vi "face rotate F+.vi"(8 "error in (no error)":errorcluster, 11 "cube in":T1) -> (0 "error out":errorcluster, 3 "cube out":T1)   [LabVIEW 2011]
uses:
  Typedef/cube.ctl
  Typedef/face.ctl
  Typedef/slice type.ctl
  Typedef/face rotate direction.ctl
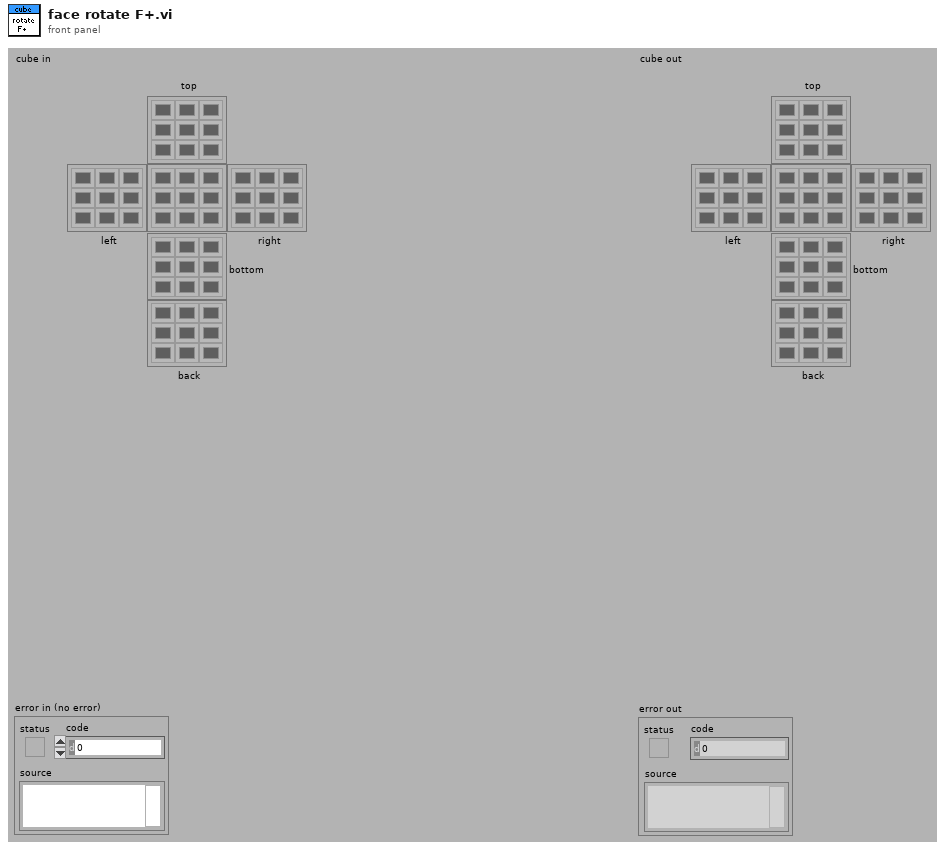
[diagram p1: front panel]
types:
  T1 = typedef "cube.ctl" = cluster{"top":T2, "left":T2, "right":T2, "bottom":T2, "back":T2, "front":T2}
  T2 = typedef "face.ctl" = u32[][]
  T3 = typedef "face rotate direction.ctl" = enum16{"+", "-"}
  T4 = typedef "slice type.ctl" = enum16{"row", "col"}
  T5 = typedef "slice.ctl" = u32[]
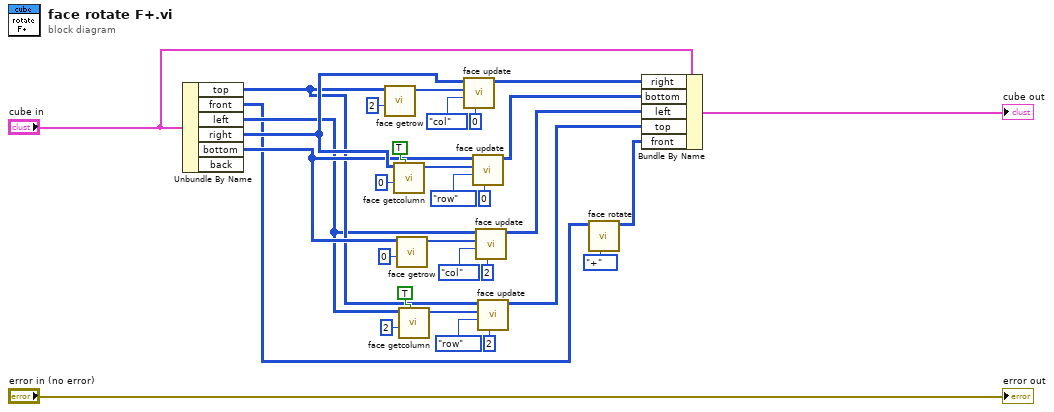
[diagram p0: block diagram]
diagram:
  n1 = Unbundle By Name("cube in") -> ("top"=w9:T2, "front"=w6:T2, "left"=w8:T2, "right"=w24:T2, "bottom"=w16:T2)  [unwired: 1 out]
  n2 = call "face getrow.vi"("row number"=u8 2, "face in"=w9) -> ("slice"=w30:T5)  [unwired: 8 in, 1 out]
  n3 = call "face getcolumn.vi"("reverse? (F)"=TRUE, "slice number"=u8 0 ("row number"), "face in"=w24) -> ("slice"=w22:T5)  [unwired: 7 in, 1 out]
  n4 = call "face getrow.vi"("row number"=u8 0, "face in"=w16) -> ("slice"=w20:T5)  [unwired: 8 in, 1 out]
  n5 = call "face getcolumn.vi"("reverse? (F)"=TRUE, "slice number"=u8 2 ("row number"), "face in"=w8) -> ("slice"=w10:T5)  [unwired: 7 in, 1 out]
  n6 = call "face update.vi"("slice number"=u8 0, "slice type"=slice_type."col", "slice"=w30, "face in"=w24) -> ("face out"=w32:T2)  [unwired: 6 in, 1 out]
  n7 = call "face update.vi"("slice number"=u8 0, "slice type"=slice_type."row", "slice"=w22, "face in"=w16) -> ("face out"=w21:T2)  [unwired: 6 in, 1 out]
  n8 = call "face update.vi"("slice number"=u8 2, "slice type"=slice_type."col", "slice"=w20, "face in"=w8) -> ("face out"=w15:T2)  [unwired: 6 in, 1 out]
  n9 = call "face update.vi"("slice number"=u8 2, "slice type"=slice_type."row", "slice"=w10, "face in"=w9) -> ("face out"=w7:T2)  [unwired: 6 in, 1 out]
  n10 = call "face rotate.vi"("rotation directon"=face_rotate_direction."+", "face in"=w6) -> ("face out"=w4:T2)  [unwired: 8 in, 1 out]
  n11 = Bundle By Name(cluster="cube in", "right"=w32, "bottom"=w21, "left"=w15, "top"=w7, "front"=w4) -> (→"cube out":T1)
  "error out" <- "error in (no error)"
